vi "Config File Path.vi"(8 "error in":errorcluster) -> (0 "error out":errorcluster, 3 "Config File Path":path)   [LabVIEW 2013, in "LVTM.lvlib"]
uses:
  LVTM.lvlib
  <vilib>/Utility/sysdir.llb/System Directory Type.ctl
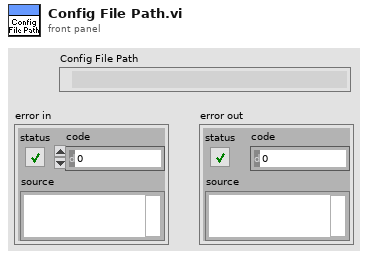
[diagram p1: front panel]
types:
  T1 = typedef "System Directory Type.ctl" = i32
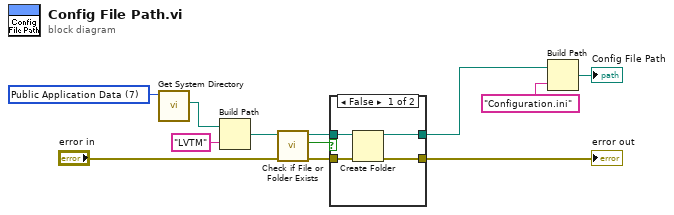
[diagram p0: block diagram]
diagram:
  w5 = T1 7 items=["User Home"=0, "User Desktop"=1, "User Documents"=2, "User Application Data"=3, "User Preferences"=4, "User Temporary"=5, "Public Documents"=6, "Public Application Data"=7, "Public Preferences"=8, "Public Cache"=13, "System Core Libraries"=9, "System Installed Libraries"=10, "Application Files"=11, "Boot Volume Root"=12] ("system directory type")
  n1 = call <vilib>:"Get System Directory.vi"("system directory type"=w5) -> ("system directory"=w6:path)  [unwired: 10 in]
  n2 = Build Path(base path=w6, name or relative path="LVTM") -> (appended path=w8:path)
  n3 = call <vilib>:"Check if File or Folder Exists.vi"("error in (no error)"="error in", "path"=w8) -> ("error out"=w2:errorcluster, "file or folder exists?"=w1:bool, "dup path"=w10:path)  [unwired: 7 in]
  n4 = case shown="False" w1 {
    tunnel: w10 -> [w16 w18]
    tunnel: [w15 w18] -> w4
    tunnel: [w14 w17] -> w3
    tunnel: w2 -> [w13 w17]
    frame False {
      n5 = Create Folder(path (use dialog)=w16, error in=w13) -> (created path=w15:path, error out=w14:errorcluster)  [unwired: 1 in, 1 out]
    }
    frame True {
    }
  }
  "error out" <- w3
  n6 = Build Path(base path=w4, name or relative path="Configuration.ini") -> (appended path=→"Config File Path":path)
